vi "counter 1.vi"() -> (0 "Counter 1":i32 caption="Zählwert 1")   [LabVIEW 2023]
doc: "The first counter. Can be run without main.vi with counter 2"
uses:
  cntrls/control_enum.ctl
panel:
  in  "Stop":bool
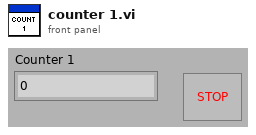
[diagram p1: front panel]
types:
  T1 = typedef "control_enum.ctl" = enum16{"read", "write", "clear"}
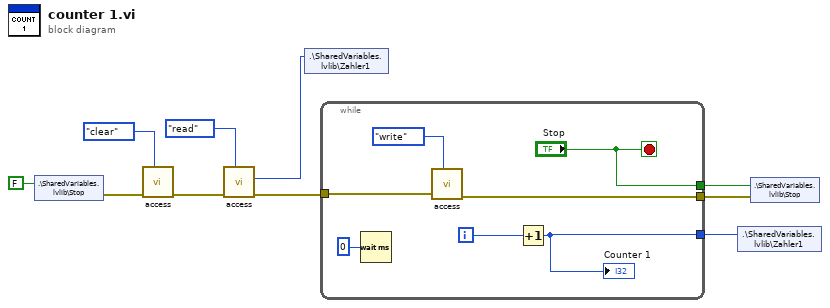
[diagram p0: block diagram]
diagram:
  n1 = shared-variable ".\\SharedVariables.lvlib\\Stop"(FALSE ("stop")) -> (error out=w5:errorcluster)  [unwired: 1 in]
  n2 = call "access.vi"("Control_enum"=control_enum."clear", "error in (no error)"=w5) -> ("error out"=w3:errorcluster)  [unwired: 6 in, 1 out]
  n3 = call "access.vi"("Control_enum"=control_enum."read", "error in (no error)"=w3) -> ("error out"=w2:errorcluster, "output"=w1:u32)  [unwired: 6 in]
  n4 = shared-variable ".\\SharedVariables.lvlib\\Zahler1"(w1) -> ()  [unwired: 1 in, 1 out]
  n5 = while {
    tunnel: w2 -> [w12]
    tunnel: [w15] -> w9
    tunnel: ["Stop"] -> w8
    tunnel: [w13] -> w7
    i -> [w14]
    stop <- "Stop" stop-if-true
    n6 = Wait (ms)(milliseconds to wait=u32 0) -> ()  [unwired: 1 out]
    n7 = call "access.vi"("Control_enum"=control_enum."write", "error in (no error)"=w12) -> ("error out"=w15:errorcluster)  [unwired: 6 in, 1 out]
    n8 = Increment(x=w14) -> (x+1=w13:i32)
    "Counter 1" <- w13
  }
  n9 = shared-variable ".\\SharedVariables.lvlib\\Zahler1"(w7) -> ()  [unwired: 1 in, 1 out]
  n10 = shared-variable ".\\SharedVariables.lvlib\\Stop"(w8, error in=w9) -> ()  [unwired: 1 out]
